vi "p2.vi"() -> ()   [LabVIEW 2021, in "d1.lvlib"]
uses:
  d1.lvlib
  AOC/AOC.lvlib
panel:
  in  "Example":string="1000\n2000\n3000\n\n4000\n\n5000\n6000\n\n7000\n8000\n9000\n\n10000\n"
  in  "Example?":bool
  out "Answer":i32=211447
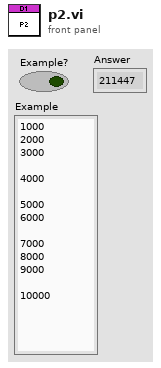
[diagram p1: front panel]
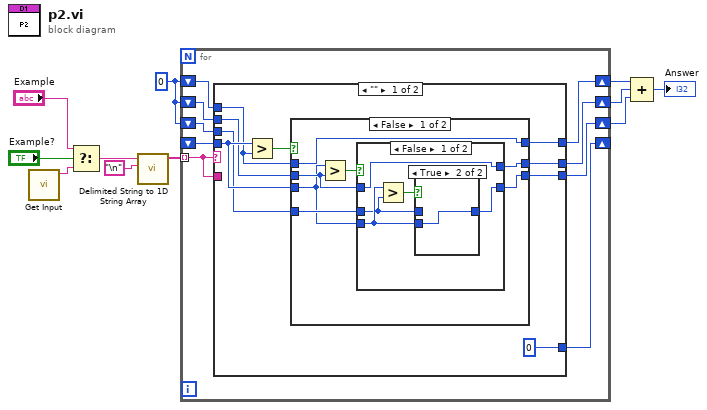
[diagram p0: block diagram]
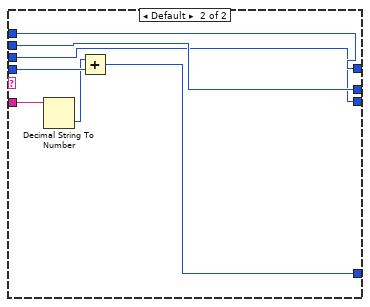
[diagram p5: hidden frame]
diagram:
  w11 = 0
  n1 = call "Get Input.vi"() -> ("Input"=w5:string)  [unwired: 11 in]
  n2 = Select(t="Example", s="Example?", f=w5) -> (s? t:f=w3:string)
  n3 = call <vilib>:"Delimited String to 1D String Array.vi"("delimiter"="\n", "delimited string"=w3) -> ("string array"=w1:string[])  [unwired: 9 in]
  n4 = for {
    tunnel: w1 -> [w18] mode=indexing
    shift-right: [w20] -> _
    shift-left: _ -> [w19]
    shift-right: [w17] -> w9
    shift-left: w11 -> [w16]
    shift-right: [w13] -> w10
    shift-left: w11 -> [w15]
    shift-right: [w12] -> w8
    shift-left: w11 -> [w14]
    n5 = case shown="\"\"" w18 {
      tunnel: [0 w55] -> w20
      tunnel: w19 -> [w26 w54]
      tunnel: w18 -> [_ w52]
      tunnel: [w28 w51] -> w17
      tunnel: w16 -> [w25 w51]
      tunnel: w15 -> [w24 w50]
      tunnel: w14 -> [w23 w49]
      tunnel: [w22 w50] -> w13
      tunnel: [w21 w49] -> w12
      frame "" {
        n6 = Greater?(x=w26, y=w25) -> (0:w27:bool)
        n7 = case shown="False" w27 {
          tunnel: [w32 w48] -> w28
          tunnel: w26 -> [w33 w48]
          tunnel: w25 -> [w32 w47]
          tunnel: w24 -> [w34 w46]
          tunnel: w23 -> [w35 _]
          tunnel: [w31 w47] -> w22
          tunnel: [w30 w46] -> w21
          frame False {
            n8 = Greater?(x=w33, y=w34) -> (0:w36:bool)
            n9 = case shown="False" w36 {
              tunnel: w35 -> [w37 _]
              tunnel: w34 -> [w39 w44]
              tunnel: w33 -> [w40 w45]
              tunnel: [w39 w45] -> w31
              tunnel: [w38 w44] -> w30
              frame False {
                n10 = Greater?(x=w40, y=w37) -> (0:w41:bool)
                n11 = case shown="True" w41 {
                  tunnel: w40 -> [_ w43]
                  tunnel: [w42 w43] -> w38
                  tunnel: w37 -> [w42 _]
                  frame False {
                  }
                  frame True {
                  }
                }
              }
              frame True {
              }
            }
          }
          frame True {
          }
        }
      }
      frame Default {
        n12 = Decimal String To Number(string=w52) -> (number=w53:i32)  [unwired: 2 in, 1 out]
        n13 = Add(x=w53, y=w54) -> (x+y=w55:i32)
      }
    }
  }
  n14 = Compound Arithmetic op=ADD(w9, w10, w8) -> (→"Answer":i32)
